vi "DATABothPDs.vi"(7 "loops x measure":i32=10, 8 "error in 2":errorcluster, 9 "error in 1":errorcluster, 10 "Visa Ref in 2":refnum<visa-resource-name> caption="instrument handle", 11 "Visa Ref in 1":refnum<visa-resource-name> caption="instrument handle") -> (0 "error out 2":errorcluster, 1 "error out 1":errorcluster, 2 "Visa ref out2":refnum<visa-resource-name>, 3 "Visa ref out 1":refnum<visa-resource-name>, 4 "Power 2":dbl format="%_7g", 5 "Transmittance PD 1/2":dbl, 6 "Power":dbl format="%_7g")   [LabVIEW 2018]
uses:
  <vilib>/Analysis/baseanly.llb/Mean (DBL).vi
  <vilib>/Analysis/NI_AALBase.lvlib
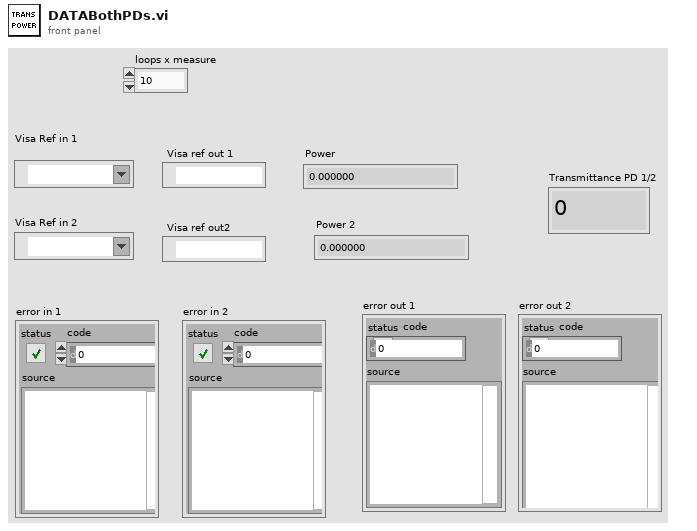
[diagram p1: front panel]
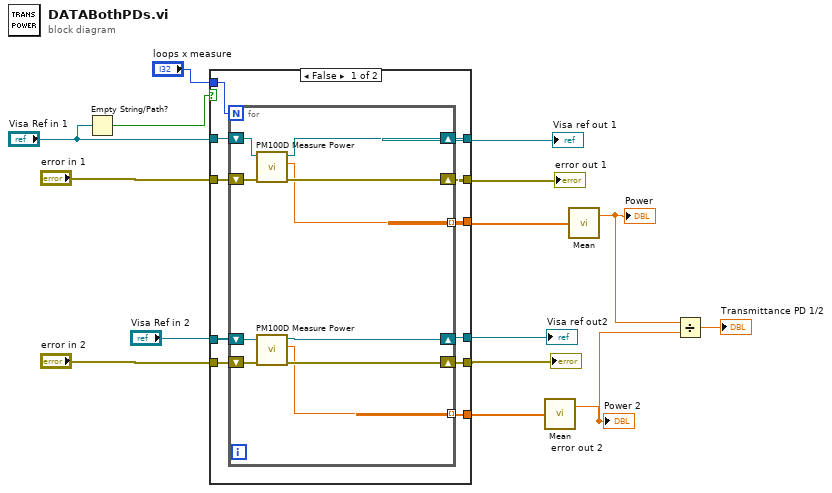
[diagram p0: block diagram]
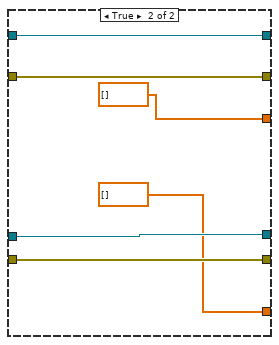
[diagram p2: hidden frame]
diagram:
  n1 = Empty String/Path?(string/path="Visa Ref in 1") -> (empty?=w15:bool)
  n2 = case shown="False" w15 {
    tunnel: "loops x measure" -> [w26 _]
    tunnel: [w25 w41] -> w11
    tunnel: [w24 w40] -> w10
    tunnel: [w23 dbl[] []] -> w13
    tunnel: "Visa Ref in 1" -> [w22 w41]
    tunnel: "error in 1" -> [w21 w40]
    tunnel: "error in 2" -> [w20 w38]
    tunnel: "Visa Ref in 2" -> [w19 w39]
    tunnel: [w18 w38] -> w6
    tunnel: [w17 w39] -> w5
    tunnel: [w16 dbl[] []] -> w4
    frame False {
      n3 = for {
        N: w26 -> [_]
        shift-right: [w34] -> w25
        shift-left: w22 -> [w36]
        shift-right: [w33] -> w24
        shift-left: w21 -> [w35]
        tunnel: [w32] -> w23 mode=indexing
        shift-right: [w28] -> w17
        shift-left: w19 -> [w30]
        shift-right: [w29] -> w18
        shift-left: w20 -> [w31]
        tunnel: [w27] -> w16 mode=indexing
        n4 = call "PM100D Measure Power.vi"("error in (no error)"=w35, "instrument handle"=w36) -> ("error out"=w33:errorcluster, "Power"=w32:dbl, "instrument handle out"=w34:refnum<visa-resource-name>)  [unwired: 7 in]
        n5 = call "PM100D Measure Power.vi"("error in (no error)"=w31, "instrument handle"=w30) -> ("error out"=w29:errorcluster, "Power"=w27:dbl, "instrument handle out"=w28:refnum<visa-resource-name>)  [unwired: 7 in]
      }
    }
    frame True {
    }
  }
  "Visa ref out 1" <- w11
  "error out 1" <- w10
  "Visa ref out2" <- w5
  "error out 2" <- w6
  n6 = call-poly <vilib>:"Mean.vi"("X"=w4) -> ("mean"=w2:dbl)  [unwired: 1 out]
  "Power 2" <- w2
  n7 = call-poly <vilib>:"Mean.vi"("X"=w13) -> ("mean"=w3:dbl)  [unwired: 1 out]
  "Power" <- w3
  n8 = Divide(x=w3, y=w2) -> (x/y=→"Transmittance PD 1/2":dbl)
